vi "TestMainPage.vi"() -> ()   [LabVIEW 2013]
uses:
  GlobalStop.vi
panel:
  out "number (0 to 1)":dbl
  out "VI Name":string
  in  "stop":bool
  in  "page2":bool
  in  "page1":bool
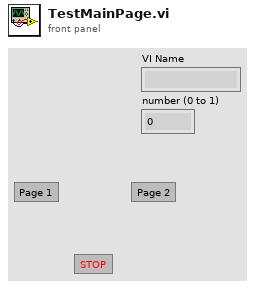
[diagram p1: front panel]
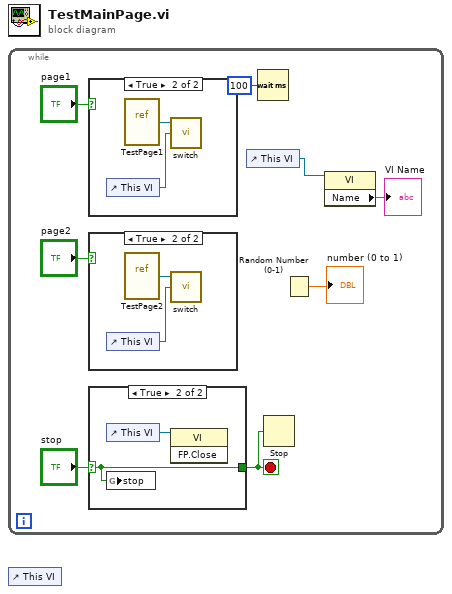
[diagram p0: block diagram]
diagram:
  n1 = while {
    stop <- w5 stop-if-true
    n2 = case shown="True" "page1" {
      frame False {
      }
      frame True {
        n3 = control-ref of="This VI"() -> (w13:refnum<vi>)
        n4 = vi-ref "TestPage1.vi"() -> (w14:refnum<vi>)
        n5 = call "switch.vi"("vi close"=w13, "vi open"=w14) -> ()  [unwired: 1 in, 1 out]
      }
    }
    n6 = case shown="True" "page2" {
      frame False {
      }
      frame True {
        n7 = control-ref of="This VI"() -> (w11:refnum<vi>)
        n8 = vi-ref "TestPage2.vi"() -> (w12:refnum<vi>)
        n9 = call "switch.vi"("vi close"=w11, "vi open"=w12) -> ()  [unwired: 1 in, 1 out]
      }
    }
    n10 = case shown="True" "stop" {
      selector: "stop" -> [_ w9]
      tunnel: [_ w9] -> w5
      frame False {
      }
      frame True {
        n11 = control-ref of="This VI"() -> (w10:refnum<vi>)
        n12 = global write "GlobalStop.vi" "stop"(w9) -> ()
        n13 = invoke class="VI" method="FP.Close"(reference=w10) -> ()  [unwired: 2 in, 3 out]
      }
    }
    n14 = control-ref of="This VI"() -> (w3:refnum<vi>)
    n15 = Wait (ms)(milliseconds to wait=u32 100) -> ()  [unwired: 1 out]
    n16 = Stop(stop? (T)=w5) -> ()
    n17 = Random Number (0-1)() -> (number: 0 to 1=→"number (0 to 1)":dbl)
    n18 = property class="VI"(reference=w3) -> ("Name"=→"VI Name":string)  [unwired: 1 in, 2 out]
  }
  n19 = control-ref of="This VI"() -> ()  [unwired: 1 out]
